vi "Onenote_Auth_handler.vi"(8 "error in (no error)":errorcluster, 10 "Auth Time In":dbl, 11 "Paths":T2) -> (0 "error out":errorcluster, 2 "Auth Time Out":dbl, 3 "Codes":T1)   [LabVIEW 2016]
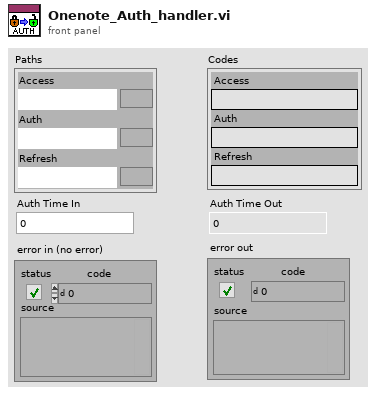
[diagram p1: front panel]
types:
  T1 = cluster{"Access":string, "Auth":string, "Refresh":string}
  T2 = cluster{"Access":path, "Auth":path, "Refresh":path}
  T3 = enum16{"open", "replace", "create", "open or create", "replace or create", "replace or create with confirmation"}
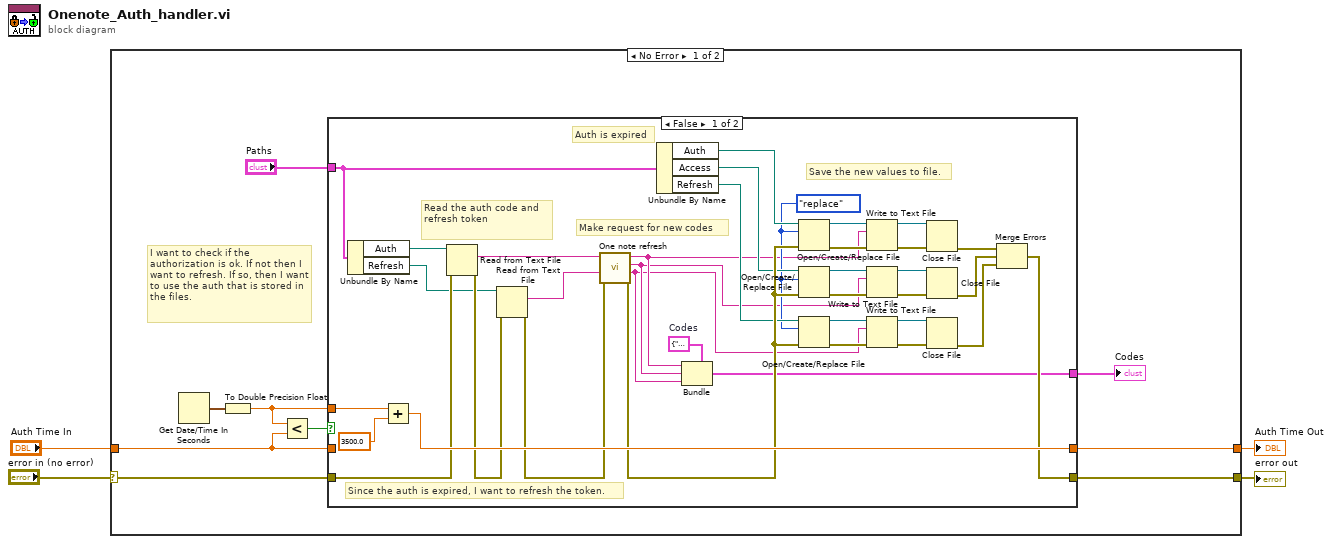
[diagram p0: block diagram]
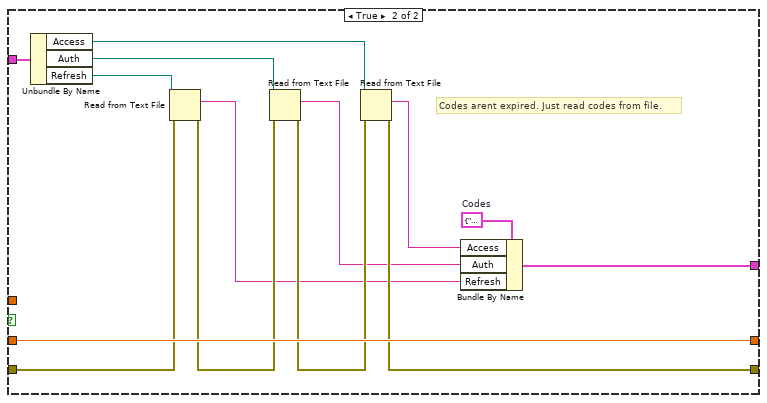
[diagram p2: hidden frame]
diagram:
  n1 = case shown="No Error" "error in (no error)" {
    selector: "error in (no error)" -> [w9 w66]
    tunnel: [w8 w66] -> w3
    tunnel: "Auth Time In" -> [w7 w65]
    tunnel: [w6 w65] -> w1
    frame No Error {
      # "I want to check if the authorization is ok. If not then I want to refresh. If so, then I want to use the auth that is stored in the files."
      n2 = Get Date/Time In Seconds() -> (seconds since 1Jan1904=w13:timestamp)
      n3 = To Double Precision Float(number=w13) -> (double precision float=w11:dbl)
      n4 = Less?(x=w11, y=w7) -> (x < y?=w12:bool)
      n5 = case shown="False" w12 {
        tunnel: w7 -> [_ w64]
        tunnel: w11 -> [w50 _]
        tunnel: [w48 w64] -> w6
        tunnel: "Paths" -> [w32 w63]
        tunnel: w9 -> [w37 w59]
        tunnel: [w23 w56] -> w8
        tunnel: [w18 w52] -> w5
        frame False {
          w19 = T3."replace" ("operation (0:open)")
          w17 = T1 {"Access"="", "Auth"="", "Refresh"=""}  # Codes
          # "Save the new values to file."
          # "Make request for new codes"
          # "Read the auth code and refresh token"
          # "Auth is expired"
          # "Since the auth is expired, I want to refresh the token."
          n6 = Unbundle By Name(w32) -> ("Auth"=w47:path, "Refresh"=w34:path)
          n7 = Add(x=w50, y=3500.0) -> (x+y=w48:dbl)
          n8 = Read from Text File(file (use dialog)=w47, error in=w37) -> (text=w46:string, error out=w36:errorcluster)  [unwired: 2 in, 2 out]
          n9 = Read from Text File(file (use dialog)=w34, error in=w36) -> (text=w35:string, error out=w33:errorcluster)  [unwired: 2 in, 2 out]
          n10 = call "One note refresh.vi"("error in (no error)"=w33, "Refresh Token In"=w35, "Authorization Code In"=w46) -> ("error out"=w24:errorcluster, "Refresh Token Out"=w14:string, "Access Token Out"=w15:string, "Authorization Code Out"=w16:string)  [unwired: 5 in]
          n11 = Unbundle By Name(w32) -> ("Auth"=w22:path, "Access"=w21:path, "Refresh"=w20:path)
          n12 = Bundle(cluster=w17, "Access"=w16, "Auth"=w15, "Refresh"=w14) -> (w18:T1)
          n13 = Open/Create/Replace File(file path (use dialog)=w22, error in=w24, operation (0:open)=w19) -> (refnum out=w38:refnum<file>, error out=w40:errorcluster)  [unwired: 3 in, 1 out]
          n14 = Open/Create/Replace File(file path (use dialog)=w21, error in=w24, operation (0:open)=w19) -> (refnum out=w45:refnum<file>, error out=w43:errorcluster)  [unwired: 3 in, 1 out]
          n15 = Open/Create/Replace File(file path (use dialog)=w20, error in=w24, operation (0:open)=w19) -> (refnum out=w28:refnum<file>, error out=w30:errorcluster)  [unwired: 3 in, 1 out]
          n16 = Write to Text File(file (use dialog)=w38, text=w16, error in=w40) -> (refnum out=w39:refnum<file>, error out=w41:errorcluster)  [unwired: 1 in, 1 out]
          n17 = Write to Text File(file (use dialog)=w45, text=w15, error in=w43) -> (refnum out=w44:refnum<file>, error out=w42:errorcluster)  [unwired: 1 in, 1 out]
          n18 = Write to Text File(file (use dialog)=w28, text=w14, error in=w30) -> (refnum out=w29:refnum<file>, error out=w31:errorcluster)  [unwired: 1 in, 1 out]
          n19 = Close File(refnum=w39, error in=w41) -> (error out=w27:errorcluster)  [unwired: 1 out]
          n20 = Close File(refnum=w44, error in=w42) -> (error out=w26:errorcluster)  [unwired: 1 out]
          n21 = Close File(refnum=w29, error in=w31) -> (error out=w25:errorcluster)  [unwired: 1 out]
          n22 = Merge Errors(w27, w26, w25) -> (w23:errorcluster)
        }
        frame True {
          w51 = T1 {"Access"="", "Auth"="", "Refresh"=""}  # Codes
          # "Codes arent expired. Just read codes from file."
          n23 = Unbundle By Name(w63) -> ("Access"=w62:path, "Auth"=w61:path, "Refresh"=w60:path)
          n24 = Read from Text File(file (use dialog)=w60, error in=w59) -> (text=w54:string, error out=w58:errorcluster)  [unwired: 2 in, 2 out]
          n25 = Read from Text File(file (use dialog)=w61, error in=w58) -> (text=w53:string, error out=w57:errorcluster)  [unwired: 2 in, 2 out]
          n26 = Read from Text File(file (use dialog)=w62, error in=w57) -> (text=w55:string, error out=w56:errorcluster)  [unwired: 2 in, 2 out]
          n27 = Bundle By Name(cluster=w51, "Access"=w55, "Auth"=w53, "Refresh"=w54) -> (w52:T1)
        }
      }
      "Codes" <- w5
    }
    frame Error {
    }
  }
  "error out" <- w3
  "Auth Time Out" <- w1
